vi "Actor Core.vi"(8 "error in":errorcluster, 11 "State Machine in":refnum<class "State Machine.lvclass">) -> (0 "error out":errorcluster, 3 "Actor out":refnum<class "Actor.lvclass">)   [LabVIEW 2024, in "State Machine.lvlib" / "State Machine.lvclass"]
doc: "<p>(<strong>Filename</strong>: <span class=\"dnl\">Actor Framework.lvlib:Actor.lvclass:Actor Core.vi</span>)</p>\n<p>Receives messages to the actor, reacts to them, and initiates any error handling that may shut the actor down.</p>\n<p>Descendant classes may override this VI to append parallel tasks for the actor to complete while it handles messages. Overrides use the <a href=\"nihelplauncher://docs/csh?context=lvcore_glang_udclass\">Call Parent Class Method</a> node.</p>"
uses:
  State Machine.lvclass
  <vilib>/ActorFramework/Actor/Actor.lvclass
  State Machine.lvclass/State Machine.ctl
  Context/Context/Context.lvclass
panel:
  out "notification":string
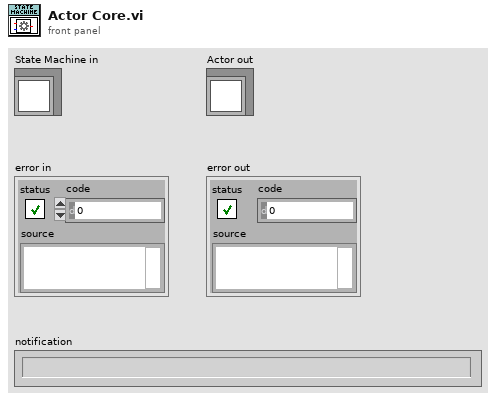
[diagram p1: front panel]
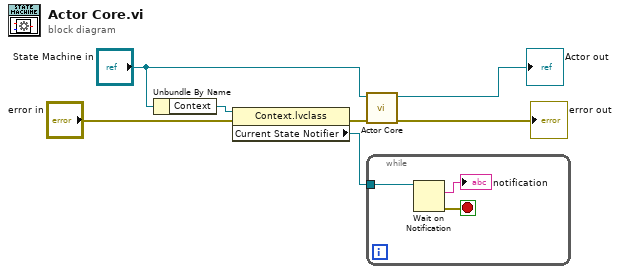
[diagram p0: block diagram]
diagram:
  n1 = Unbundle By Name("State Machine in") -> ("Context"=w4:refnum<class "Context.lvclass">)
  n2 = property class="Context.lvclass"(reference=w4, error in="error in") -> (error out=w1:errorcluster, "Current State Notifier"=w3:refnum<notifier>)  [unwired: 1 out]
  n3 = call-parent "Actor Core.vi"("error in"=w1, "Actor in"="State Machine in") -> ("error out"=→"error out":errorcluster, "Actor out"=→"Actor out":refnum<class "Actor.lvclass">)  [unwired: 8 in]
  n4 = while {
    tunnel: w3 -> [w10]
    stop <- w9 stop-if-true
    n5 = Wait on Notification(notifier=w10) -> (notification=→"notification":string, error out=w9:errorcluster)  [unwired: 3 in, 2 out]
  }
